vi "SL TAGS Set Value By Name.vi"(4 "Tag Scope":T1=enum."Server", 6 "Tag Type":T2, 8 "error in (no error)":errorcluster, 9 "Value":variant, 10 "Tag Name":string, 11 "EEISysLink in":refnum<class "EEISysLink.lvclass">) -> (0 "error out":errorcluster, 3 "EEISysLink out":refnum<class "EEISysLink.lvclass">)   [LabVIEW 2017, in "EEISysLink.lvclass"]
doc: "Will update the current value of the first tag that matches the input name. \n\nJames Tillett P.E.\nEndeavor Engineering Inc.\nwww.endeavoreng.com"
uses:
  EEISysLink.lvclass
  Controls/SL Tag Type.ctl
  Controls/SL Tag Scope.ctl
  EEISysLink.lvclass/EEISysLink.ctl
panel:
  out "Found?":bool
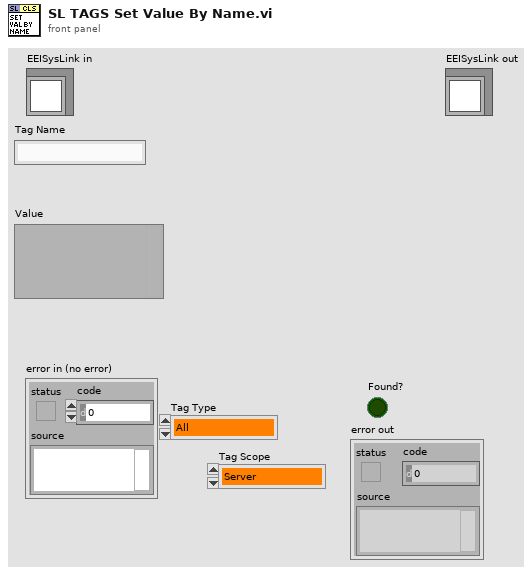
[diagram p1: front panel]
types:
  T1 = typedef "EEISysLink.lvclass/SL Tag Scope.ctl" = enum16{"Local", "Server"}
  T2 = typedef "EEISysLink.lvclass/SL Tag Type.ctl" = enum16{"All", "Supervisor", "Worker"}
  T3 = typedef "EEISysLink.lvclass/SL Tag.ctl" = cluster{"Class Properties":T4, "SL Tag":refnum<class "NI Skyline Tag.lvclass">, "SystemLink Cluster":T8, "Class Value":variant}
  T4 = typedef "EEISysLink.lvclass/SL Tag Properties.ctl" = cluster{"Class Data Type":T5, "Name":string, "Description":string, "Interpolation Method":T6, "Unit of Measure":T7, "Maximum Interpolation":string, "Role":T2}
  T5 = typedef "EEISysLink.lvclass/SL Tag Data Type.ctl" = enum16{"Double", "Integer", "String", "Boolean", "Waveform"}
  T6 = typedef "EEISysLink.lvclass/SL Tag Interpolation Method.ctl" = enum16{"linear", "pilinear", "step"}
  T7 = typedef "EEISysLink.lvclass/SL Tag Unit of Measure.ctl" = enum16{"no units", "Second", "Hour", "Minute", "Day", "Year", "Month", "Week", "Foot", "Yard", "Meter", "Centimeter", "Inch", "Mile", "Nautical Mile", "Miles per Hour", "Meters per second", "Square meter", "Cubic meter", "Cubic centimeter", "Cubic inch", "Liter", "Gallon", "Gallons dry US", "Gallon UK", "Percent", "Revolutions per minute", "Revolution", "Degree angle", "Astronomical Unit", "Atom", "Atomic mass", "Bar", "Byte", "C (speed of light)", "Curie", "Decibel", "Electron Volt", "Ounce", "Knot", "G", "Grade", "Are", "Hectare", "Faraday", "Franklin", "Gilbert", "Erg", "Lambert", "Maxwell", "Gauss", "Electron mass", "Kilogram force", "Pound force", "Rad", "Centiradian", "Sphere", "Mach", "Fluid Ounces", "Fluid Ounces UK", "Fahrenheit", "Celsius", "Kelvin", "Rankine", "Gram", "Kilogram", "Pound", "Short/US Ton", "Long/UK ton", "Metric ton", "Mole", "Pounds per square inch", "Inches water column", "Torr", "Millitorr", "Millimeter mercury", "Inches mercury", "Bar (2)", "Atmosphere", "Pascal", "Watt", "kiloWatt", "Horsepower", "Kilowatt Hour", "British thermal units", "Millions of BTU", "Ampere", "Candela", "Radian", "Steradian", "Bit", "Hertz", "Newton", "Joule", "Coulomb", "Volt", "Farad", "Ohm", "Siemens", "Weber", "Tesla", "Henry", "Lumen", "Lux", "Becqueral", "Gray", "Sievert", "Katal", "Angstrom", "Light Year", "Parsec", "Point", "Pixel", "Dyne", "Kilogram force (2)", "Pound force (2)", "Rem", "Rutherford", "Roentgen"}
  T8 = typedef "NI Skyline Tag.lvlib/Tag Cluster.ctl" = cluster{"Path":string, "Data Type":T9, "Value":variant, "Time Stamp":timestamp}
  T9 = typedef "NI Skyline Tag.lvlib/DataType.ctl" = enum32{"Double", "Integer", "String"}
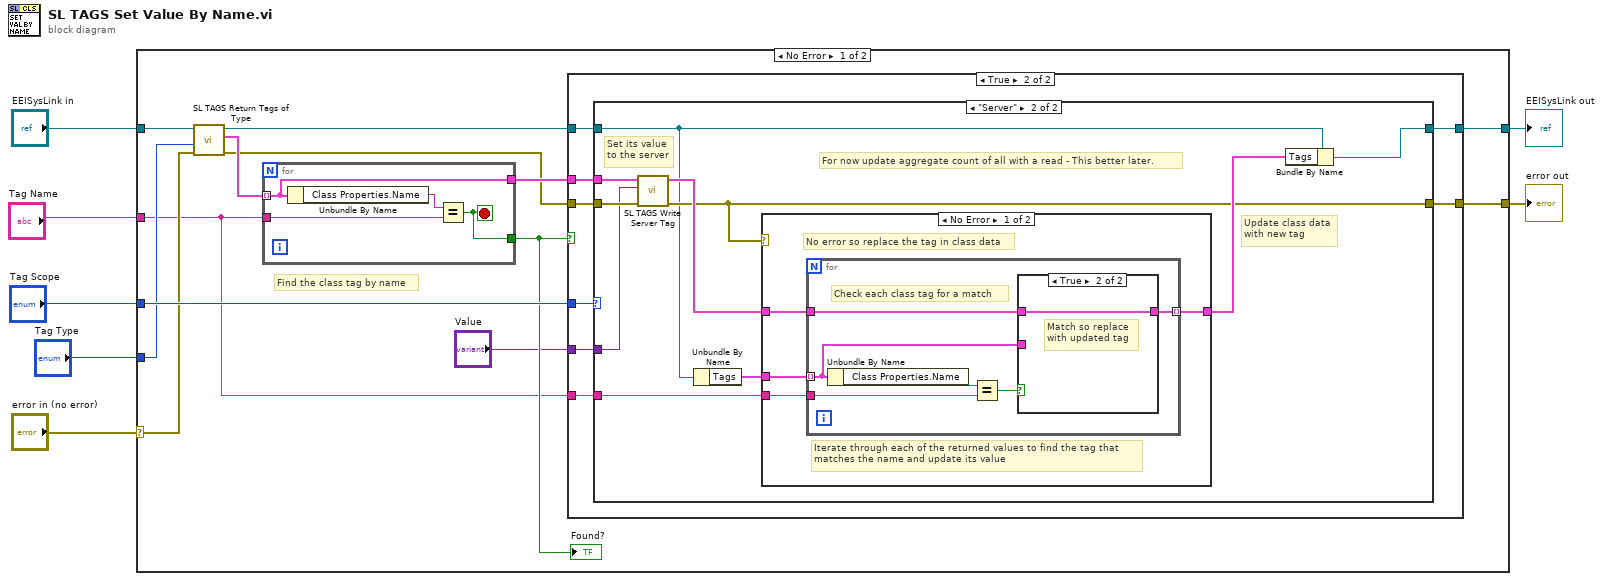
[diagram p0: block diagram]
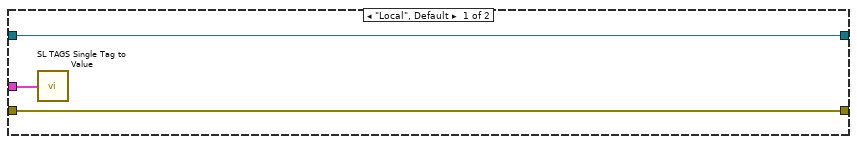
[diagram p3: hidden frame]
diagram:
  n1 = case shown="No Error" "error in (no error)" {
    selector: "error in (no error)" -> [w15 w62]
    tunnel: [w9 w62] -> w6
    tunnel: [w19 w61] -> w4
    tunnel: "EEISysLink in" -> [w18 w61]
    tunnel: "Tag Scope" -> [w20 _]
    tunnel: "Tag Type" -> [w14 _]
    tunnel: "Tag Name" -> [w11 _]
    frame No Error {
      # "Find the class tag by name"
      n2 = call "SL TAGS Return Tags of Type.vi"("error in (no error)"=w15, "Tag Type"=w14, "EEISysLink in"=w18) -> ("error out"=w10:errorcluster, "Tags of Type"=w16:T3[], "EEISysLink out"=w17:refnum<class "EEISysLink.lvclass">)  [unwired: 6 in]
      n3 = for {
        tunnel: w16 -> [w58] mode=indexing
        tunnel: w11 -> [w60]
        tunnel: [w58] -> w12
        tunnel: [w57] -> w13
        stop <- w57 stop-if-true
        n4 = Unbundle By Name(w58) -> ("Class Properties.Name"=w59:string)
        n5 = Equal?(x=w59, y=w60) -> (x = y?=w57:bool)
      }
      "Found?" <- w13
      n6 = case shown="True" w13 {
        tunnel: w20 -> [_ w30]
        tunnel: [w22 w29] -> w19
        tunnel: w17 -> [w22 w28]
        tunnel: w12 -> [_ w27]
        tunnel: w11 -> [_ w26]
        tunnel: w10 -> [w21 w25]
        tunnel: [w21 w24] -> w9
        tunnel: "Value" -> [_ w23]
        frame False {
          # "Tag not found"
        }
        frame True {
          n7 = case shown="\"Server\"" w30 {
            tunnel: w28 -> [w33 w35]
            tunnel: [w33 w42] -> w29
            tunnel: w27 -> [w32 w40]
            tunnel: w26 -> [_ w39]
            tunnel: w25 -> [w31 w37]
            tunnel: [w31 w36] -> w24
            tunnel: w23 -> [_ w34]
            frame "Local", Default {
              n8 = call "SL TAGS Single Tag to Value.vi"("Tag"=w32) -> ()  [unwired: 4 in, 1 out]
            }
            frame "Server" {
              # "For now update aggregate count of all with a read - This better later."
              # "Set its value\nto the server"
              # "Update class data\nwith new tag"
              n9 = call "SL TAGS Write Server Tag.vi"("error in (no error)"=w37, "Value"=w34, "Tag Ref In"=w40) -> ("error out"=w36:errorcluster, "Tag Ref Out"=w38:T3)  [unwired: 7 in]
              n10 = Unbundle By Name(w35) -> ("Tags"=w43:T3[])
              n11 = case shown="No Error" w36 {
                tunnel: w43 -> [w47 w56]
                tunnel: [w46 w56] -> w41
                tunnel: w39 -> [w45 _]
                tunnel: w38 -> [w44 _]
                frame No Error {
                  # "Iterate through each of the returned values to find the tag that\nmatches the name and update its value"
                  # "No error so replace the tag in class data"
                  n12 = for {
                    tunnel: w47 -> [w50] mode=indexing
                    tunnel: w44 -> [w51]
                    tunnel: [w49] -> w46 mode=indexing
                    tunnel: w45 -> [w48]
                    # "Check each class tag for a match"
                    n13 = Unbundle By Name(w50) -> ("Class Properties.Name"=w53:string)
                    n14 = Equal?(x=w53, y=w48) -> (x = y?=w52:bool)
                    n15 = case shown="True" w52 {
                      tunnel: w51 -> [_ w55]
                      tunnel: w50 -> [w54 _]
                      tunnel: [w54 w55] -> w49
                      frame False {
                        # "Names don't match\nso do nothing"
                      }
                      frame True {
                        # "Match so replace\nwith updated tag"
                      }
                    }
                  }
                }
                frame Error {
                  # "Error on update so don't change tag values"
                }
              }
              n16 = Bundle By Name(cluster=w35, "Tags"=w41) -> (w42:refnum<class "EEISysLink.lvclass">)
            }
          }
        }
      }
    }
    frame Error {
    }
  }
  "error out" <- w6
  "EEISysLink out" <- w4
